vi "Top-Level VI_2014.vi"(0 "sequenceFilePath":string="C:\\Teststand\\Teststand_Main_v3.seq") -> ()   [LabVIEW 2014]
doc: "This is the main VI in the TestStand Simple User Interface."
uses:
  Engine/TestExec.llb/State Selector.ctl
  Engine/TestExec.llb/TestStand UI Data.ctl
  SharedVariables/TSE_Variables.vi
  Engine/TestExec.llb/TestStand Simple UI Dependencies.lvlib
panel:
  out "GetItemText":string
  out "Executing":bool
  in  "Start":bool
  in  "Terminate All Button":refnum<k7>(container)
  in  "Exit Button":refnum<k7>(container)
  in  "Login/Logout Button":refnum<k7>(container)
  in  "Close Executions Button":refnum<k7>(container)
  in  "Break/Resume Button":refnum<k7>(container)
  in  "Terminate/Restart Button":refnum<k7>(container)
  in  "Run Selected Sequence Button":refnum<k7>(container)
  in  "Entry Point 2 Button":refnum<k7>(container)
  in  "Entry Point 1 Button":refnum<k7>(container)
  in  "Report Viewer":refnum<k7>(container)
  in  "Close Sequence File Button":refnum<k7>(container)
  in  "Open Sequence File Button":refnum<k7>(container)
  in  "Executions ComboBox":refnum<k7>(container) caption="Executions:"
  in  "Sequences ComboBox":refnum<k7>(container) caption="Sequences:"
  in  "Execution View":refnum<k7>(container)
  in  "Sequence Files ComboBox":refnum<k7>(container) caption="Sequence Files:"
  in  "ExecutionView Manager":refnum<k7>(container)
  in  "SequenceFileView Manager":refnum<k7>(container)
  in  "Application Manager":refnum<k7>(container)
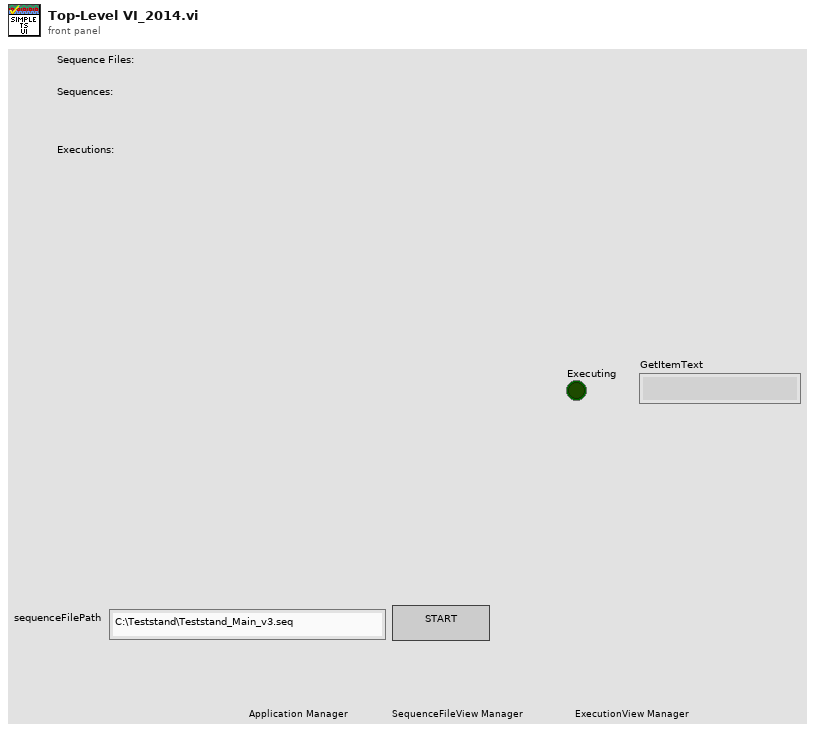
[diagram p1: front panel]
types:
  T1 = typedef "TestStand Simple UI Dependencies.lvlib/TestStand UI Data.ctl" = cluster{"Other References":cluster{"Event Callback":refnum<k27>, "Quit Application Event":refnum<user-event>, "Event Reg Refnum":refnum<event-registration>, "Top level VI":refnum<vi>, "TestStand Engine":refnum<k7>}, "Manager Controls":cluster{"Application Manager":refnum<k7>, "SequenceFileView Manager":refnum<k7>, "ExecutionView Manager":refnum<k7>}, "Visible Controls":cluster{"Terminate/Restart Button":refnum<k7>, "Break/Resume Button":refnum<k7>, "Close Executions Button":refnum<k7>, "Report Viewer":refnum<k7>, "Execution View":refnum<k7>, "Executions ComboBox":refnum<k7>, "Run Selected Sequence Button":refnum<k7>, "Entry Point 2 Button":refnum<k7>, "Entry Point 1 Button":refnum<k7>, "Close Sequence File Button":refnum<k7>, "Open Sequence File Button":refnum<k7>, "Sequences ComboBox":refnum<k7>, "Sequence Files ComboBox":refnum<k7>, "Terminate All Button":refnum<k7>, "Exit Button":refnum<k7>, "Login/Logout Button":refnum<k7>}}
  T2 = typedef "TestStand Simple UI Dependencies.lvlib/State Selector.ctl" = enum16{"Initialize", "Configure Connections", "Register Event Callbacks", "Start Application", "Handle Events", "Shutdown", "Handle Errors"}
  T3 = enum32{"invalid app kind", "Development System", "Run Time System", "Student Edition", "Embedded LabVIEW", "Evaluation", "Custom"}
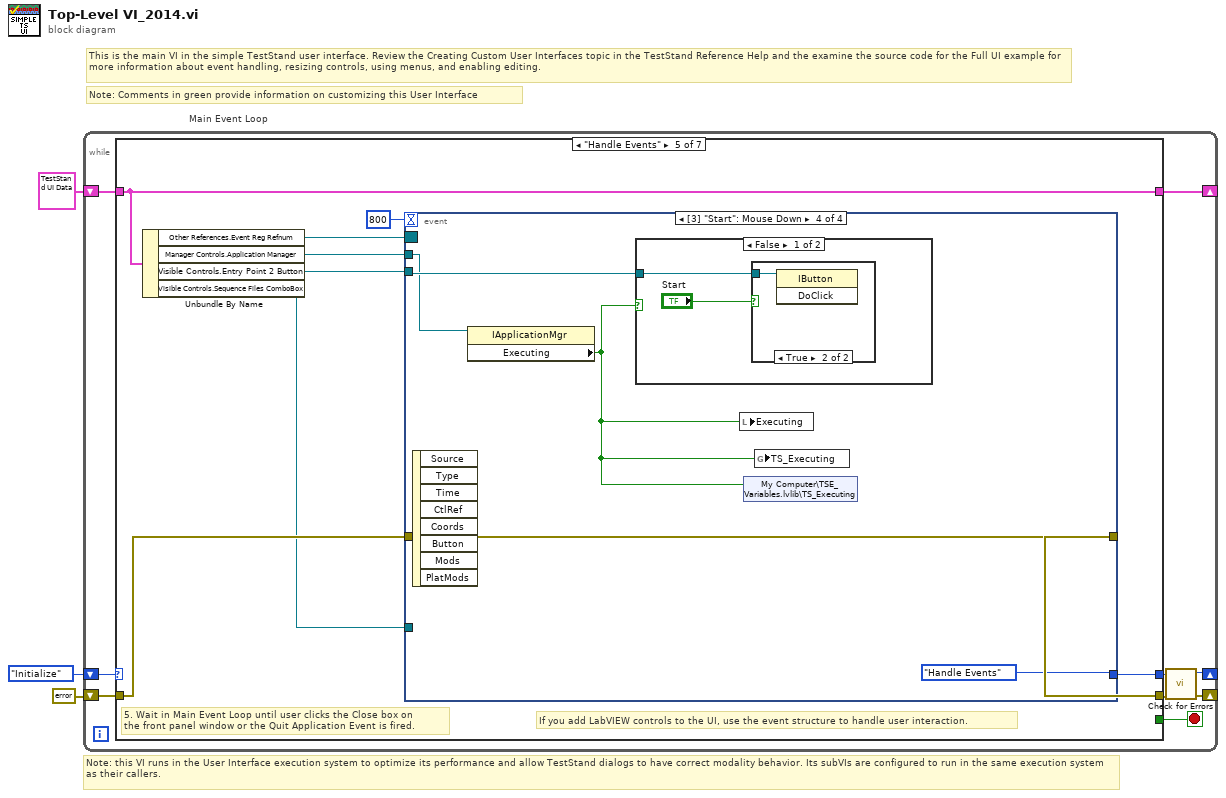
[diagram p0: block diagram]
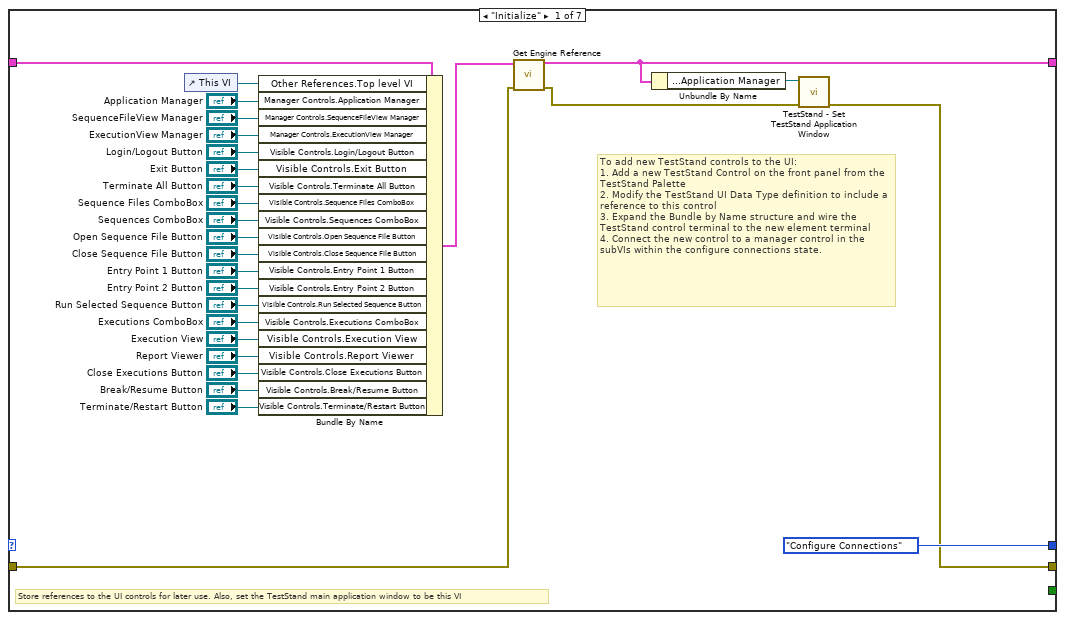
[diagram p2: hidden frame]
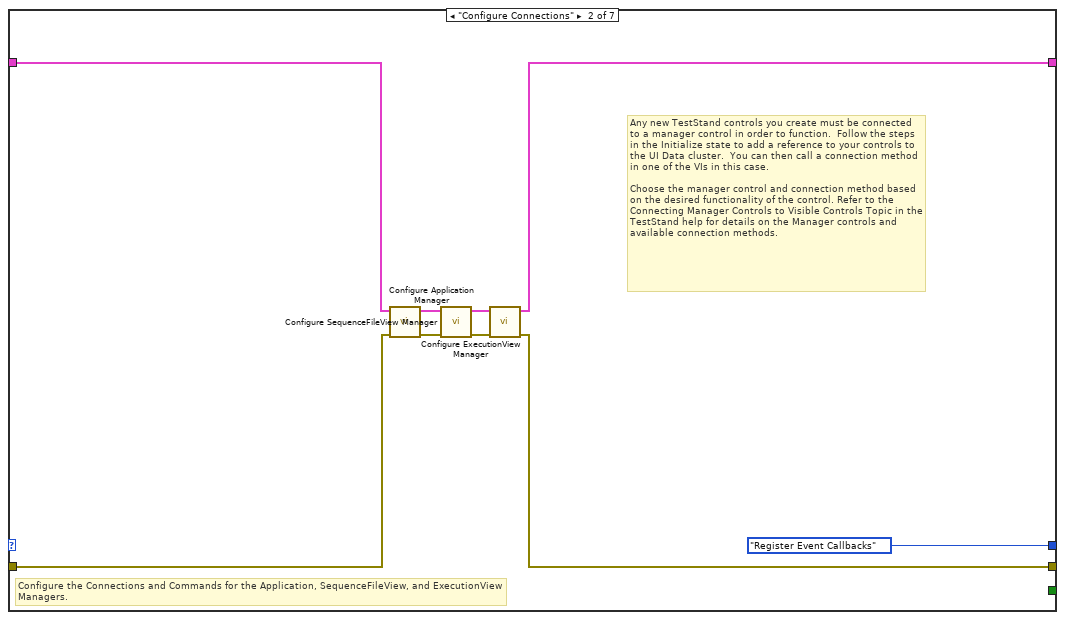
[diagram p3: hidden frame]
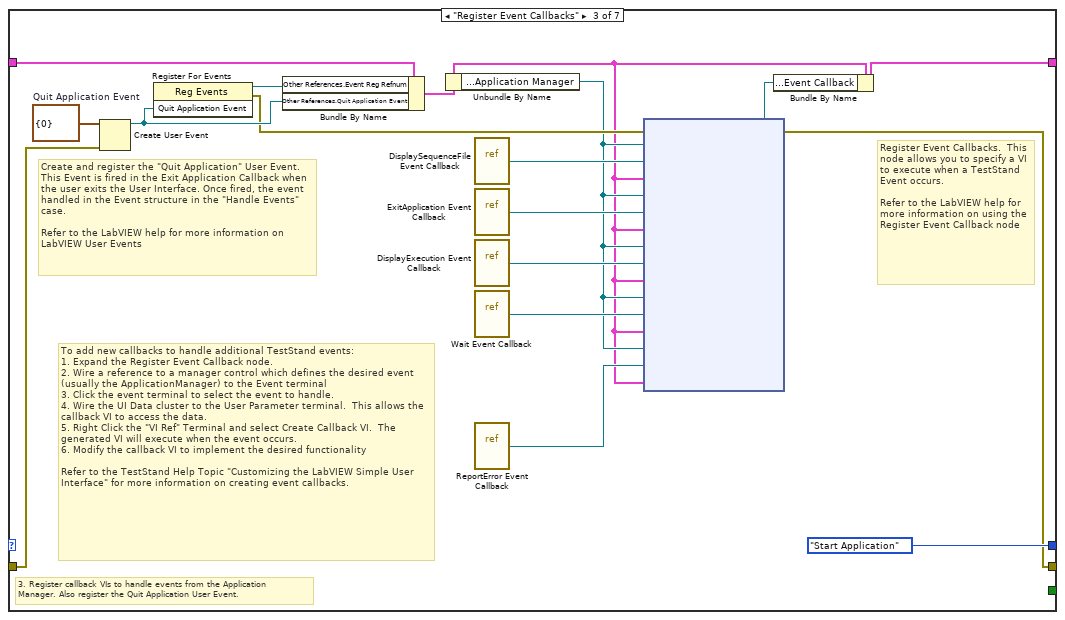
[diagram p4: hidden frame]
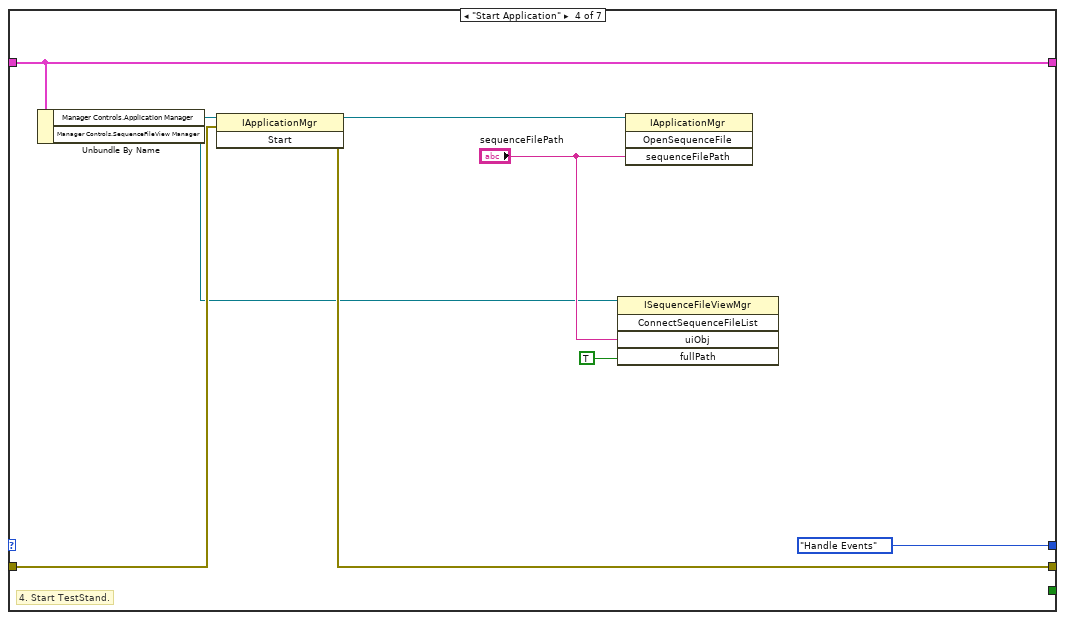
[diagram p5: hidden frame]
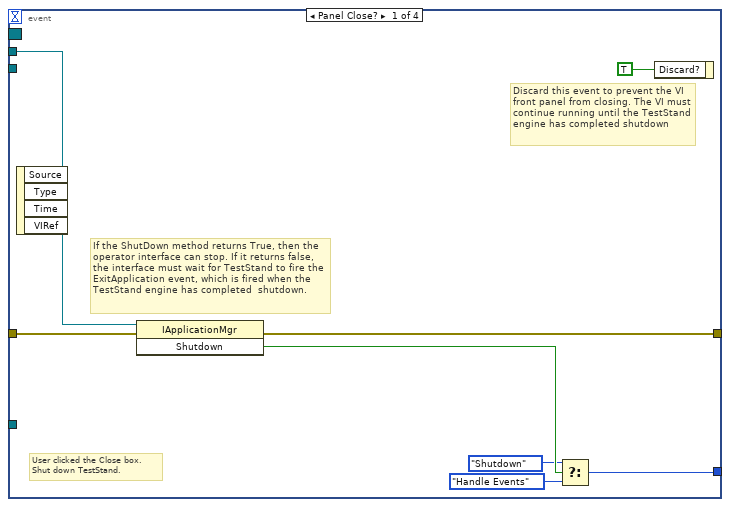
[diagram p6: hidden frame]
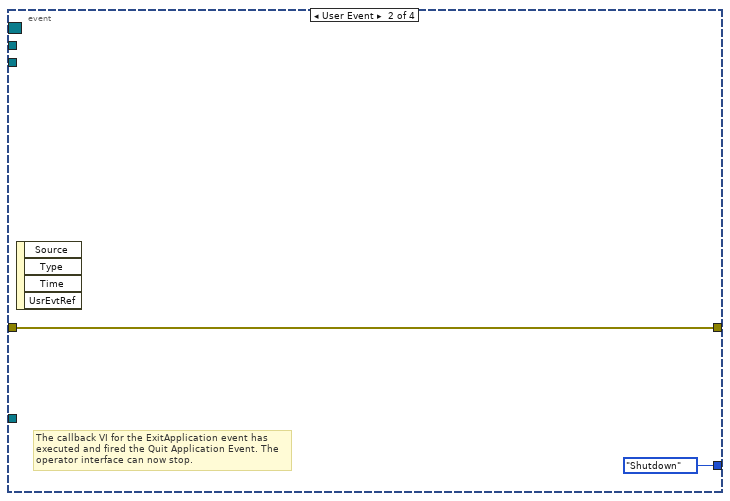
[diagram p7: hidden frame]
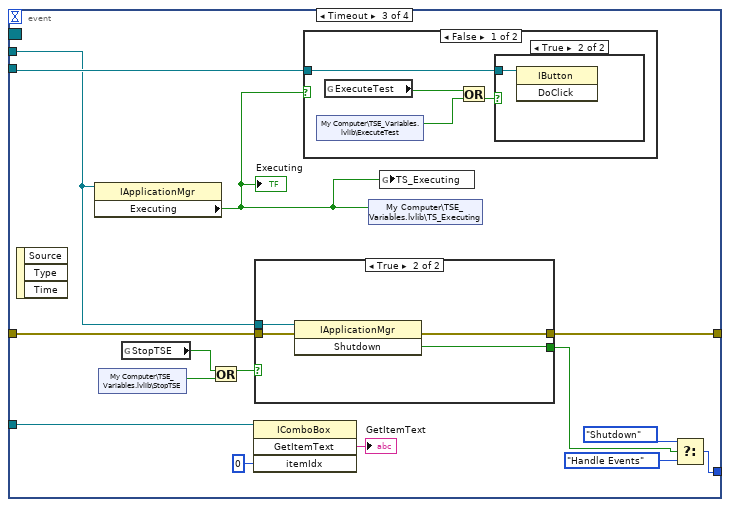
[diagram p8: hidden frame]
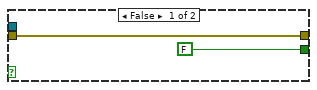
[diagram p11: hidden frame]
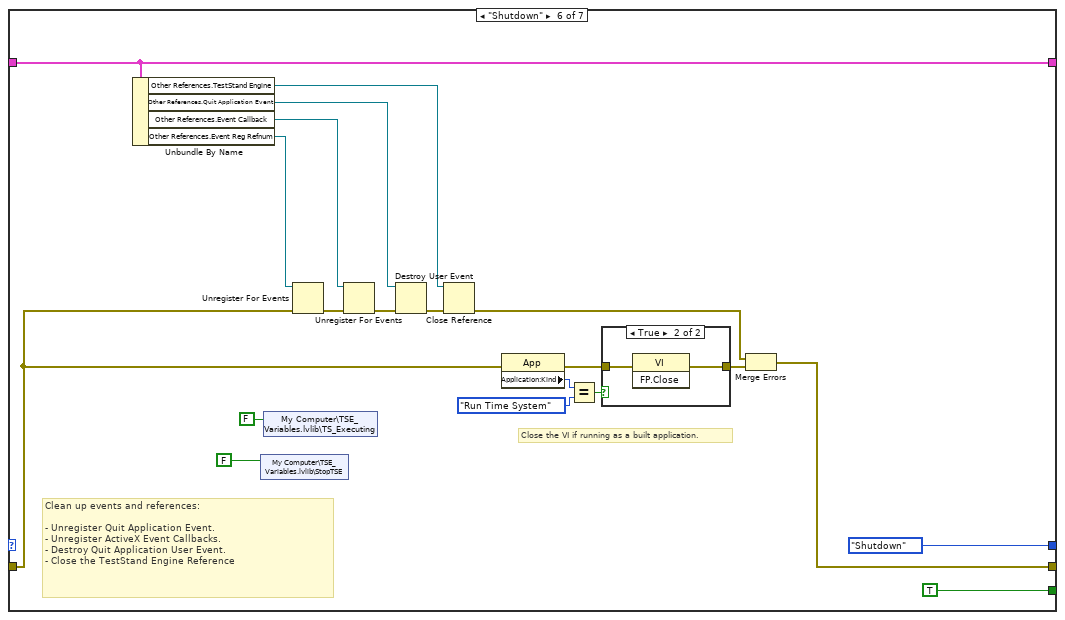
[diagram p14: hidden frame]
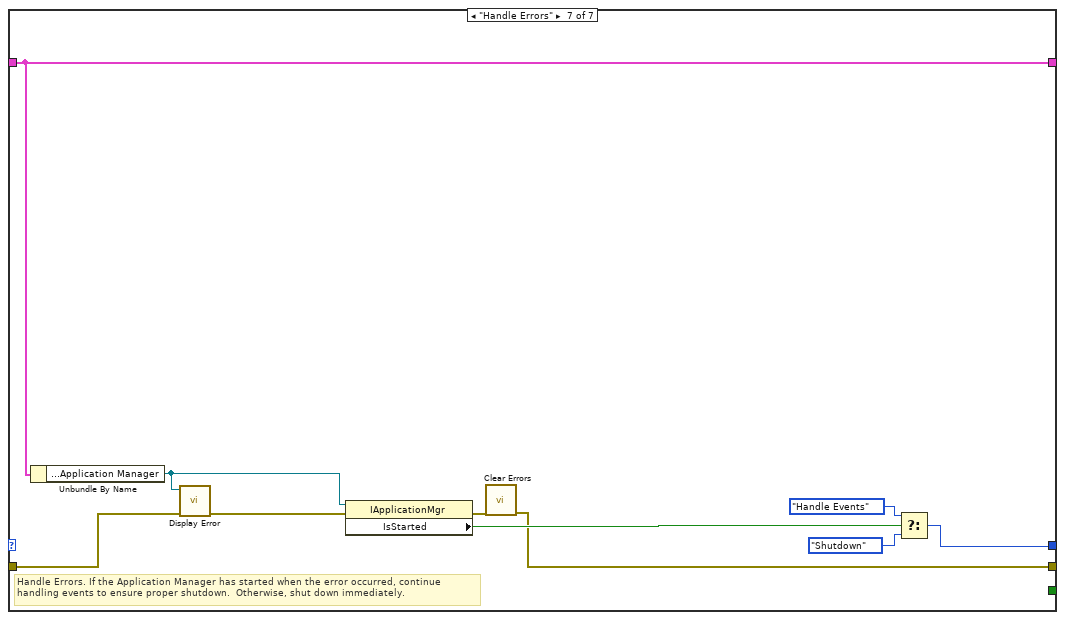
[diagram p16: hidden frame]
diagram:
  # "Note: Comments in green provide information on customizing this User Interface"
  # "Note: this VI runs in the User Interface execution system to optimize its performance and allow TestStand dialogs to have correct modality behavior. Its subVIs are configured to run in the same execution system as their callers."
  # "This is the main VI in the simple TestStand user interface. Review the Creating Custom User Interfaces topic in the TestStand Reference Help and the examine the source code for the Full UI example for more information about event handling, resizing controls, using menus, and enabling editing."
  n1 = while "Main Event Loop" {
    shift-right: [w5] -> _
    shift-left: errorcluster {"status"=FALSE, "code"=0, "source"=""} ("error out") -> [w12]
    shift-right: [w6] -> _
    shift-left: State_Selector."Initialize" ("Enum") -> [w9]
    shift-right: [w11] -> _
    shift-left: T1 {"Other References"={"Event Callback"=refnum, "Quit Application Event"=refnum, "Event Reg Refnum"=refnum, "Top level VI"=refnum, "TestStand Engine"=refnum}, "Manager Controls"={"Application Manager"=refnum, "SequenceFileView Manager"=refnum, "ExecutionView Manager"=refnum}, "Visible Controls"={"Terminate/Restart Button"=refnum, "Break/Resume Button"=refnum, "Close Executions Button"=refnum, "Report Viewer"=refnum, "Execution View"=refnum, "Executions ComboBox"=refnum, "Run Selected Sequence Button"=refnum, "Entry Point 2 Button"=refnum, "Entry Point 1 Button"=refnum, "Close Sequence File Button"=refnum, "Open Sequence File Button"=refnum, "Sequences ComboBox"=refnum, "Sequence Files ComboBox"=refnum, "Terminate All Button"=refnum, "Exit Button"=refnum, "Login/Logout Button"=refnum}} ("TestStand UI Data") -> [w10]
    stop <- w8 stop-if-true
    n2 = case shown="\"Handle Events\"" w9 {
      tunnel: w12 -> [w21 w41 w65 w73 w84 w134 w161]
      tunnel: [w17 w47 w52 w72 w80 w131 w152] -> w4
      tunnel: [w19 w42 w63 w75 w83 w143 w160] -> w11
      tunnel: w10 -> [w15 w43 w54 w75 w83 w143 w160]
      tunnel: [State_Selector."Configure Connections" ("Enum") State_Selector."Register Event Callbacks" ("Enum") State_Selector."Start Application" ("Enum") State_Selector."Handle Events" ("Enum") w82 State_Selector."Shutdown" ("Enum") w154] -> w7
      tunnel: [_ _ _ _ _ TRUE ("ShutDown") _] -> w8
      frame "Initialize" {
        # "To add new TestStand controls to the UI:\n1. Add a new TestStand Control on the front panel from the TestStand Palette \n2. Modify the TestStand UI Data Type definition to include a reference to this control\n3. Expand the Bundle by Name structure and wire the TestStand control terminal to the new element terminal\n4. Connect the new control to a manager control in the subVIs within the configure connections state."
        # "Store references to the UI controls for later use. Also, set the TestStand main application window to be this VI"
        n3 = control-ref of="This VI"() -> (w23:refnum<vi>)
        n4 = Bundle By Name(cluster=w15, "Other References.Top level VI"=w23, "Manager Controls.Application Manager"="Application Manager", "Manager Controls.SequenceFileView Manager"="SequenceFileView Manager", "Manager Controls.ExecutionView Manager"="ExecutionView Manager", "Visible Controls.Login/Logout Button"="Login/Logout Button", "Visible Controls.Exit Button"="Exit Button", "Visible Controls.Terminate All Button"="Terminate All Button", "Visible Controls.Sequence Files ComboBox"="Sequence Files ComboBox", "Visible Controls.Sequences ComboBox"="Sequences ComboBox", "Visible Controls.Open Sequence File Button"="Open Sequence File Button", "Visible Controls.Close Sequence File Button"="Close Sequence File Button", "Visible Controls.Entry Point 1 Button"="Entry Point 1 Button", "Visible Controls.Entry Point 2 Button"="Entry Point 2 Button", "Visible Controls.Run Selected Sequence Button"="Run Selected Sequence Button", "Visible Controls.Executions ComboBox"="Executions ComboBox", "Visible Controls.Execution View"="Execution View", "Visible Controls.Report Viewer"="Report Viewer", "Visible Controls.Close Executions Button"="Close Executions Button", "Visible Controls.Break/Resume Button"="Break/Resume Button", "Visible Controls.Terminate/Restart Button"="Terminate/Restart Button") -> (w14:T1)
        n5 = call "Get Engine Reference.vi"("error in (no error)"=w21, "TestStand UI Data In"=w14) -> ("error out"=w18:errorcluster, "TestStand UI Data Out"=w19:T1)  [unwired: 8 in]
        n6 = Unbundle By Name(w19) -> ("Manager Controls.Application Manager"=w20:refnum<k7>)
        n7 = call <vilib>:"TestStand - Set TestStand Application Window.vi"("error in (no error)"=w18, "Application Manager"=w20) -> ("error out"=w17:errorcluster)  [unwired: 1 in, 8 out]
      }
      frame "Configure Connections" {
        # "Any new TestStand controls you create must be connected to a manager control in order to function.  Follow the steps in the Initialize state to add a reference to your controls to the UI Data cluster.  You can then call a connection method in one of the VIs in this case.  \n\nChoose the manager control and connection method based on the desired functionality of the control. Refer to the Connecting Manager Controls to Visible Controls Topic in the TestStand help for details on the Manager controls and available connection methods."
        # "Configure the Connections and Commands for the Application, SequenceFileView, and ExecutionView Managers."
        n8 = call "Configure Application Manager.vi"("error in (no error)"=w41, "TestStand Controls"=w43) -> ("error out"=w49:errorcluster, "TestStand Controls Out"=w45:T1)  [unwired: 1 in, 7 out]
        n9 = call "Configure SequenceFileView Manager.vi"("error in (no error)"=w49, "TestStand Controls"=w45) -> ("error out"=w48:errorcluster, "TestStand Controls Out"=w44:T1)  [unwired: 8 in]
        n10 = call "Configure ExecutionView Manager.vi"("error in (no error)"=w48, "TestStand Controls"=w44) -> ("error out"=w47:errorcluster, "TestStand Controls Out"=w42:T1)  [unwired: 6 in, 2 out]
      }
      frame "Register Event Callbacks" {
        w66 = cluster{"Number":i32} {"Number"=0}  # Quit Application Event
        # "Register Event Callbacks.  This node allows you to specify a VI to execute when a TestStand Event occurs. \n\nRefer to the LabVIEW help for more information on using the Register Event Callback node"
        # "Create and register the \"Quit Application\" User Event. This Event is fired in the Exit Application Callback when the user exits the User Interface. Once fired, the event handled in the Event structure in the \"Handle Events\" case.\n\nRefer to the LabVIEW help for more information on LabVIEW User Events"
        # "To add new callbacks to handle additional TestStand events:\n1. Expand the Register Event Callback node.  \n2. Wire a reference to a manager control which defines the desired event (usually the ApplicationManager) to the Event terminal\n3. Click the event terminal to select the event to handle.\n4. Wire the UI Data cluster to the User Parameter terminal.  This allows the callback VI to access the data.\n5. Right Click the \"VI Ref\" Terminal and select Create Callback VI.  The generated VI will execute when the event occurs.\n6. Modify the callback VI to implement the desired functionality\n\nRefer to the TestStand Help Topic \"Customizing the LabVIEW Simple User Interface\" for more information on creating event callbacks."
        # "3. Register callback VIs to handle events from the Application\nManager. Also register the Quit Application User Event."
        n11 = Create User Event(user event datatype=w66, error in=w65) -> (user event=w56:refnum<user-event>)  [unwired: 1 out]
        n12 = register-events(w56) -> (reference out=w55:refnum<event-registration>, error out=w53:errorcluster)  [unwired: 2 in]
        n13 = Bundle By Name(cluster=w54, "Other References.Event Reg Refnum"=w55, "Other References.Quit Application Event"=w56) -> (w50:T1)
        n14 = Unbundle By Name(w50) -> ("Manager Controls.Application Manager"=w51:refnum<k7>)
        n15 = vi-ref "DisplaySequenceFile Event Callback.vi"() -> ("vi reference"=w61:refnum<vi>)
        n16 = vi-ref "ExitApplication Event Callback.vi"() -> ("vi reference"=w59:refnum<vi>)
        n17 = vi-ref "DisplayExecution Event Callback.vi"() -> ("vi reference"=w58:refnum<vi>)
        n18 = vi-ref "Wait Event Callback.vi"() -> ("vi reference"=w57:refnum<vi>)
        n19 = vi-ref "ReportError Event Callback.vi"() -> ("vi reference"=w60:refnum<vi>)
        n20 = node(w53, w51, w61, w50, w51, w59, w50, w51, w58, w50, w51, w57, w50, w51, w60, w50) -> (w62:refnum<k27>, w52:errorcluster)  [unwired: 1 in]
        n21 = Bundle By Name(cluster=w50, "Other References.Event Callback"=w62) -> (w63:T1)
      }
      frame "Start Application" {
        # "4. Start TestStand."
        n22 = Unbundle By Name(w75) -> ("Manager Controls.Application Manager"=w74:refnum<k7>, "Manager Controls.SequenceFileView Manager"=w67:refnum<k7>)
        n23 = invoke class="IApplicationMgr" method="Start"(reference=w74, error in=w73) -> (reference out=w70:refnum<k7>, error out=w72:errorcluster)  [unwired: 1 in, 1 out]
        n24 = invoke class="ISequenceFileViewMgr" method="ConnectSequenceFileList"(reference=w67, "uiObj"="sequenceFilePath", "fullPath"=TRUE) -> ()  [unwired: 2 in, 5 out]
        n25 = invoke class="IApplicationMgr" method="OpenSequenceFile"(reference=w70, "sequenceFilePath"="sequenceFilePath") -> ()  [unwired: 2 in, 4 out]
      }
      frame "Handle Events" {
        # "5. Wait in Main Event Loop until user clicks the Close box on\nthe front panel window or the Quit Application Event is fired."
        # "If you add LabVIEW controls to the UI, use the event structure to handle user interaction."
        n26 = Unbundle By Name(w83) -> ("Other References.Event Reg Refnum"=w81:refnum<event-registration>, "Manager Controls.Application Manager"=w79:refnum<k7>, "Visible Controls.Entry Point 2 Button"=w78:refnum<k7>, "Visible Controls.Sequence Files ComboBox"=w77:refnum<k7>)
        n27 = event shown="[3] \"Start\": Mouse Down" {
          selector: w81 -> [_ _ _ _]
          dyn-events: _ -> [_ _ _ _]
          timeout: 800 -> [_ _ _ _]
          tunnel: w84 -> [w92 w94 w109 w124]
          tunnel: [w91 w94 w104 w124] -> w80
          tunnel: w79 -> [w89 _ w99 w122]
          tunnel: [w85 State_Selector."Shutdown" ("Enum") w105 State_Selector."Handle Events" ("Enum")] -> w82
          tunnel: w78 -> [_ _ w103 w125]
          tunnel: w77 -> [_ _ w100 _]
          event Panel Close? {
            # "Discard this event to prevent the VI front panel from closing. The VI must continue running until the TestStand engine has completed shutdown"
            # "If the ShutDown method returns True, then the operator interface can stop. If it returns false, the interface must wait for TestStand to fire the ExitApplication event, which is fired when the TestStand engine has completed  shutdown."
            # "User clicked the Close box.\nShut down TestStand."
            n28 = event-data() -> ()  [unwired: 5 out]
            n29 = invoke class="IApplicationMgr" method="Shutdown"(reference=w89, error in=w92) -> (error out=w91:errorcluster, "Shutdown"=w88:bool)  [unwired: 1 in, 1 out]
            n30 = Select(t=State_Selector."Shutdown" ("Enum"), s=w88, f=State_Selector."Handle Events" ("Enum")) -> (s? t:f=w85:T2)
            n31 = event-data("Discard?"=TRUE) -> ()  [unwired: 1 in, 1 out]
          }
          event User Event {
            # "The callback VI for the ExitApplication event has executed and fired the Quit Application Event. The operator interface can now stop."
            n32 = event-data() -> ()  [unwired: 5 out]
          }
          event Timeout {
            n33 = event-data() -> ()  [unwired: 4 out]
            n34 = property class="IApplicationMgr"(reference=w99) -> ("Executing"=w98:bool)  [unwired: 1 in, 2 out]
            "Executing" <- w98
            n35 = shared-variable "My Computer\\TSE_Variables.lvlib\\StopTSE"() -> (w96:bool)  [unwired: 1 in, 1 out]
            n36 = global read "TSE_Variables.vi" "StopTSE"() -> (w95:bool)
            n37 = Or(x=w95, y=w96) -> (x .or. y?=w97:bool)
            n38 = invoke class="IComboBox" method="GetItemText"(reference=w100, "itemIdx"=0) -> ("GetItemText"=→"GetItemText":string)  [unwired: 2 in, 3 out]
            n39 = case shown="True" w97 {
              tunnel: [w115 w117] -> w104
              tunnel: [FALSE ("Shutdown") w120] -> w106
              tunnel: w109 -> [w115 w119]
              tunnel: w99 -> [_ w118]
              frame False {
              }
              frame True {
                n40 = invoke class="IApplicationMgr" method="Shutdown"(reference=w118, error in=w119) -> (error out=w117:errorcluster, "Shutdown"=w120:bool)  [unwired: 1 in, 1 out]
              }
            }
            n41 = case shown="False" w98 {
              tunnel: w103 -> [w113 _]
              frame False {
                n42 = shared-variable "My Computer\\TSE_Variables.lvlib\\ExecuteTest"() -> (w112:bool)  [unwired: 1 in, 1 out]
                n43 = global read "TSE_Variables.vi" "ExecuteTest"() -> (w110:bool)
                n44 = Or(x=w110, y=w112) -> (x .or. y?=w111:bool)
                n45 = case shown="True" w111 {
                  tunnel: w113 -> [_ w114]
                  frame False {
                  }
                  frame True {
                    n46 = invoke class="IButton" method="DoClick"(reference=w114) -> ()  [unwired: 2 in, 3 out]
                  }
                }
              }
              frame True {
              }
            }
            n47 = shared-variable "My Computer\\TSE_Variables.lvlib\\TS_Executing"(w98) -> ()  [unwired: 1 in, 1 out]
            n48 = global write "TSE_Variables.vi" "TS_Executing"(w98) -> ()
            n49 = Select(t=State_Selector."Shutdown" ("Enum"), s=w106, f=State_Selector."Handle Events" ("Enum")) -> (s? t:f=w105:T2)
          }
          event "Start": Mouse Down {
            n50 = event-data() -> ()  [unwired: 9 out]
            n51 = property class="IApplicationMgr"(reference=w122) -> ("Executing"=w121:bool)  [unwired: 1 in, 2 out]
            n52 = case shown="False" w121 {
              tunnel: w125 -> [w127 _]
              frame False {
                n53 = case shown="True" "Start" {
                  tunnel: w127 -> [_ w128]
                  frame False {
                  }
                  frame True {
                    n54 = invoke class="IButton" method="DoClick"(reference=w128) -> ()  [unwired: 2 in, 3 out]
                  }
                }
              }
              frame True {
              }
            }
            n55 = local write "Executing"(w121) -> ()
            n56 = shared-variable "My Computer\\TSE_Variables.lvlib\\TS_Executing"(w121) -> ()  [unwired: 1 in, 1 out]
            n57 = global write "TSE_Variables.vi" "TS_Executing"(w121) -> ()
          }
        }
      }
      frame "Shutdown" {
        # "Close the VI if running as a built application."
        # "Clean up events and references:\n\n- Unregister Quit Application Event.\n- Unregister ActiveX Event Callbacks.\n- Destroy Quit Application User Event.\n- Close the TestStand Engine Reference"
        n58 = Unbundle By Name(w143) -> ("Other References.TestStand Engine"=w139:refnum<k7>, "Other References.Quit Application Event"=w141:refnum<user-event>, "Other References.Event Callback"=w144:refnum<k27>, "Other References.Event Reg Refnum"=w142:refnum<event-registration>)
        n59 = shared-variable "My Computer\\TSE_Variables.lvlib\\StopTSE"(FALSE ("StopTSE")) -> ()  [unwired: 1 in, 1 out]
        n60 = shared-variable "My Computer\\TSE_Variables.lvlib\\TS_Executing"(FALSE ("TS_Executing")) -> ()  [unwired: 1 in, 1 out]
        n61 = Unregister For Events(event registration refnum=w142, error in=w134) -> (error out=w145:errorcluster)
        n62 = Unregister For Events(event registration refnum=w144, error in=w145) -> (error out=w146:errorcluster)
        n63 = Destroy User Event(user event=w141, error in=w146) -> (error out=w140:errorcluster)
        n64 = Close Reference(reference=w139, error in (no error)=w140) -> (error out=w132:errorcluster)
        n65 = property class="App"(error in=w134) -> (error out=w135:errorcluster, "Application:Kind"=w137:T3)  [unwired: 1 in, 1 out]
        n66 = Equal?(x=w137, y=T3."Run Time System" ("Application:Kind")) -> (x = y?=w136:bool)
        n67 = case shown="True" w136 {
          tunnel: w135 -> [w149 w151]
          tunnel: [w149 w150] -> w133
          frame False {
          }
          frame True {
            n68 = invoke class="VI" method="FP.Close"(error in=w151) -> (error out=w150:errorcluster)  [unwired: 2 in, 2 out]
          }
        }
        n69 = Merge Errors(w132, w133) -> (w131:errorcluster)
      }
      frame "Handle Errors" {
        # "Handle Errors. If the Application Manager has started when the error occurred, continue handling events to ensure proper shutdown.  Otherwise, shut down immediately."
        n70 = Unbundle By Name(w160) -> ("Manager Controls.Application Manager"=w158:refnum<k7>)
        n71 = call "Display Error.vi"("error in (no error)"=w161, "Application Manager"=w158) -> ("error out"=w159:errorcluster)  [unwired: 9 out]
        n72 = property class="IApplicationMgr"(reference=w158, error in=w159) -> (error out=w153:errorcluster, "IsStarted"=w157:bool)  [unwired: 1 out]
        n73 = call <vilib>:"Clear Errors.vi"("error in (no error)"=w153) -> ("error out"=w152:errorcluster)  [unwired: 5 in, 1 out]
        n74 = Select(t=State_Selector."Handle Events" ("Enum"), s=w157, f=State_Selector."Shutdown" ("Enum")) -> (s? t:f=w154:T2)
      }
    }
    n75 = call "Check for Errors.vi"("Error In"=w4, "State"=w7) -> ("Error Out"=w5:errorcluster, "State Out"=w6:T2)  [unwired: 8 in]
  }
